vi "Reset Graph Scale.vi"(5 "WaveformChart in":refnum<vi>, 8 "Error In":errorcluster, 10 "Minimum (0)":dbl, 11 "Maximum (100)":dbl) -> (0 "error out":errorcluster)   [LabVIEW 2012]
uses:
  <vilib>/Utility/miscctls.llb/LVRangeTypeDef.ctl
panel:
  out "output cluster":T1
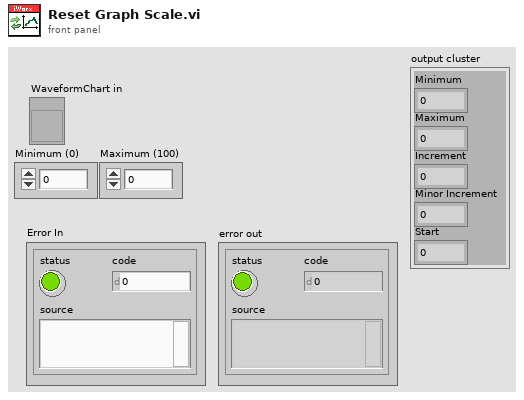
[diagram p1: front panel]
types:
  T1 = typedef "LVRangeTypeDef.ctl" = cluster{"Minimum":dbl, "Maximum":dbl, "Increment":dbl, "Minor Increment":dbl, "Start":dbl}
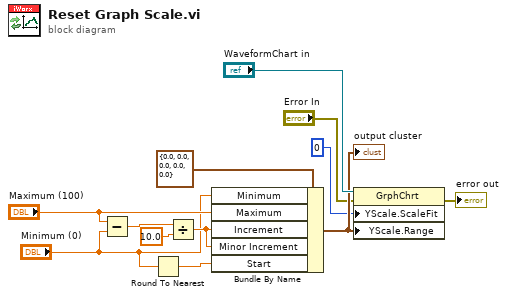
[diagram p0: block diagram]
diagram:
  n1 = Subtract(x="Maximum (100)", y="Minimum (0)") -> (x-y=w8:dbl)
  n2 = Round To Nearest(number="Minimum (0)") -> (nearest integer value=w4:dbl)
  n3 = Divide(x=w8, y=10.0) -> (x/y=w6:dbl)
  n4 = Bundle By Name(cluster=T1 {"Minimum"=0.0, "Maximum"=0.0, "Increment"=0.0, "Minor Increment"=0.0, "Start"=0.0} ("Y Scale.Range"), "Minimum"="Minimum (0)", "Maximum"="Maximum (100)", "Increment"=w6, "Minor Increment"=w6, "Start"=w4) -> (w10:T1)
  "output cluster" <- w10
  n5 = property class="GrphChrt"(reference="WaveformChart in", error in="Error In", "YScale.ScaleFit"=u8 0 ("Y Scale.Scale Fit"), "YScale.Range"=w10) -> (error out=→"error out":errorcluster)  [unwired: 1 out]
